vi "Determine Warnings .vi"() -> ()   [LabVIEW 2014]
panel:
  out "Warning Text":string
  out "Warning":bool
  in  "Min Temp":dbl
  in  "Max Temp":dbl
  in  "Current Temp":dbl
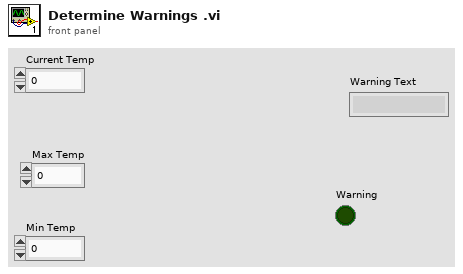
[diagram p1: front panel]
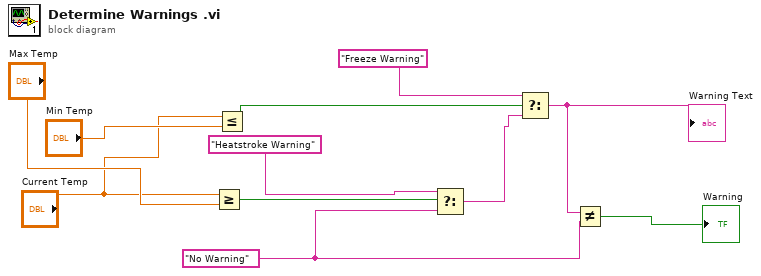
[diagram p0: block diagram]
diagram:
  w3 = "No Warning"
  n1 = Greater Or Equal?(x="Current Temp", y="Max Temp") -> (x >= y?=w9:bool)
  n2 = Less Or Equal?(x="Current Temp", y="Min Temp") -> (x <= y?=w7:bool)
  n3 = Select(t="Heatstroke Warning", s=w9, f=w3) -> (s? t:f=w5:string)
  n4 = Select(t="Freeze Warning", s=w7, f=w5) -> (s? t:f=w4:string)
  "Warning Text" <- w4
  n5 = Not Equal?(x=w4, y=w3) -> (x != y?=→"Warning":bool)
